vi "AMC_select_IP_SubVI.vi"(10 "IPs":string[](array[string]), 11 "Found Devices":T1(array[cluster])) -> (0 "error out":errorcluster, 2 "Device Info":T2, 3 "IP":string)   [LabVIEW 2019]
panel:
  out "Found devices":i32
  in  "please select IP":u16(ring) items=["10.10.1.230", "192.168.1.1"]
  in  "Refresh Button":bool
  in  "Process Stop":bool
  in  "OK Button":bool
  out "Array":T1(array[cluster])
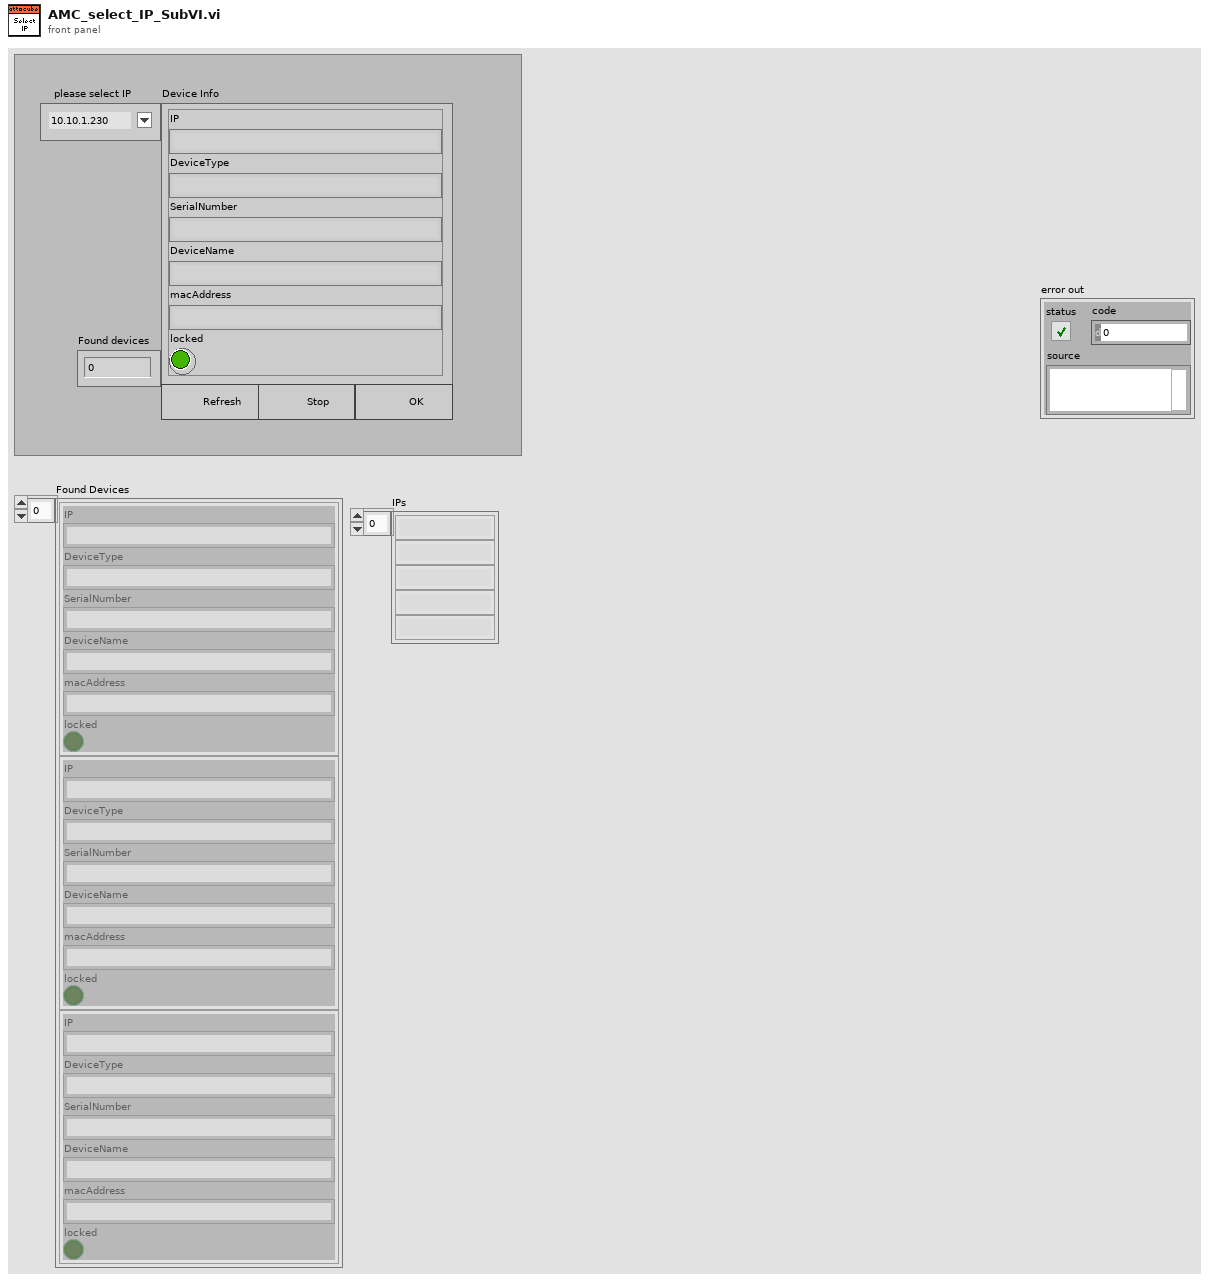
[diagram p1: front panel]
types:
  T1 = cluster{"IP":string, "DeviceType":string, "SerialNumber":string, "DeviceName":string, "macAddress":string, "locked":bool}[]
  T2 = cluster{"IP":string, "DeviceType":string, "SerialNumber":string, "DeviceName":string, "macAddress":string, "locked":bool}
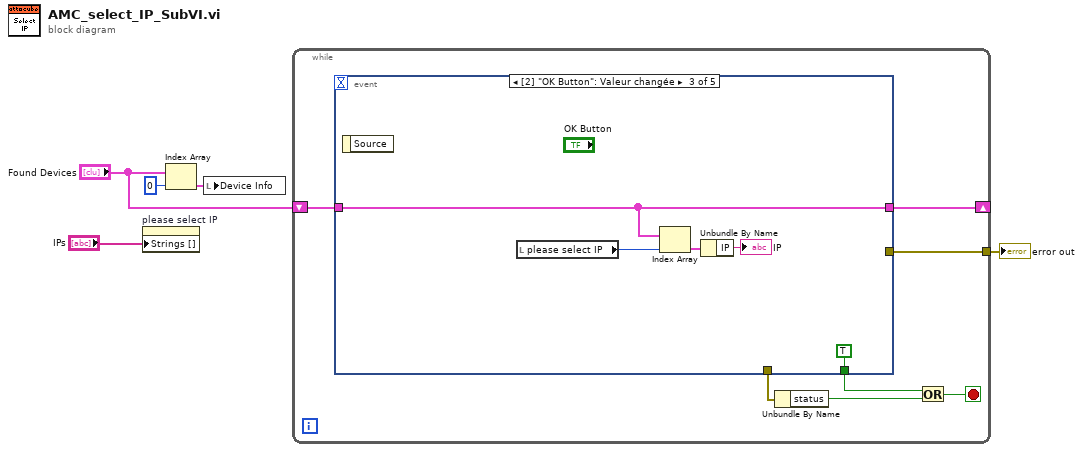
[diagram p0: block diagram]
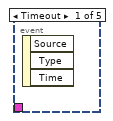
[diagram p2: hidden frame]
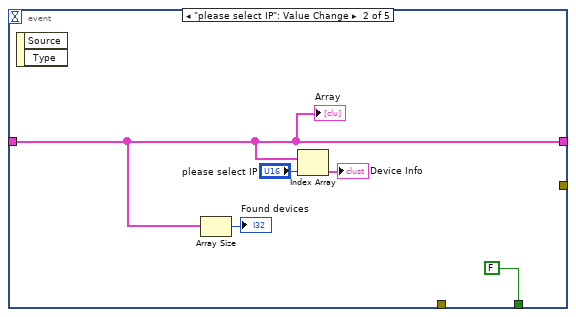
[diagram p3: hidden frame]
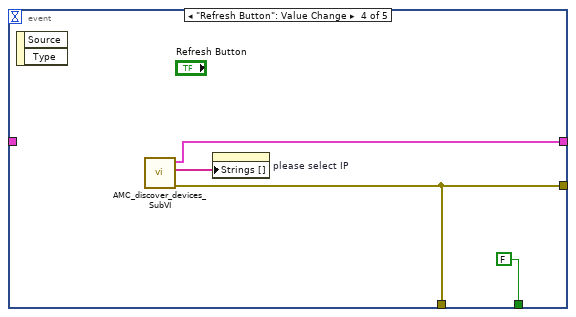
[diagram p4: hidden frame]
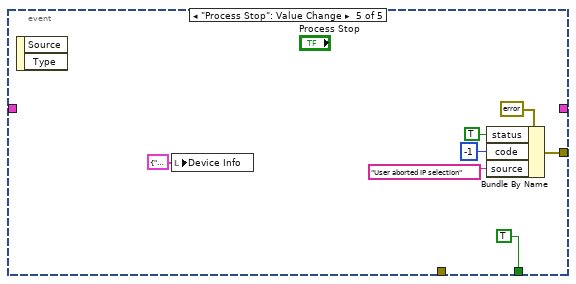
[diagram p5: hidden frame]
diagram:
  n1 = property on="please select IP" class="MDér (strict)"("Strings []"="IPs") -> ()  [unwired: 2 in, 2 out]
  n2 = Index Array(array="Found Devices", index=0) -> (element=w3:T2)
  n3 = local write "Device Info"(w3) -> ()
  n4 = while {
    shift-right: [w12] -> _
    shift-left: "Found Devices" -> [w11]
    tunnel: [w6] -> w5
    stop <- w7 stop-if-true
    n5 = event shown="[2] \"OK Button\": Valeur changée" {
      selector: _ -> [_ _ _ _ _]
      dyn-events: _ -> [_ _ _ _ _]
      timeout: _ -> [_ _ _ _ _]
      tunnel: [_ w14 w20 w25 _] -> w12
      tunnel: w11 -> [_ w14 w20 _ _]
      tunnel: [_ FALSE TRUE FALSE TRUE] -> w9
      tunnel: [_ _ _ w23 _] -> w10
      tunnel: [_ _ _ w23 w27] -> w6
      event Timeout {
        n6 = event-data() -> ()  [unwired: 1 in, 3 out]
      }
      event "please select IP": Value Change {
        n7 = event-data() -> ()  [unwired: 1 in, 2 out]
        n8 = Array Size(array=w14) -> (size(s)=→"Found devices":i32)
        n9 = Index Array(array=w14, index="please select IP") -> (element=→"Device Info":T2)
        "Array" <- w14
      }
      event "OK Button": Value Change {
        n10 = event-data() -> ()  [unwired: 1 in, 1 out]
        n11 = local read "please select IP"() -> (w18:u16)
        n12 = Index Array(array=w20, index=w18) -> (element=w21:T2)
        n13 = Unbundle By Name(w21) -> ("IP"=→"IP":string)
      }
      event "Refresh Button": Value Change {
        n14 = event-data() -> ()  [unwired: 1 in, 2 out]
        n15 = call <userlib>:"AMC_discover_devices_SubVI.vi"() -> ("error out"=w23:errorcluster, "IPs"=w26:string[], "Found Devices"=w25:T1)  [unwired: 8 in, 1 out]
        n16 = property on="please select IP" class="MDér (strict)"("Strings []"=w26) -> ()  [unwired: 2 in, 2 out]
      }
      event "Process Stop": Value Change {
        n17 = event-data() -> ()  [unwired: 1 in, 2 out]
        n18 = local write "Device Info"(T2 {"IP"="", "DeviceType"="", "SerialNumber"="", "DeviceName"="", "macAddress"="", "locked"=FALSE} ("Cluster")) -> ()
        n19 = Bundle By Name(cluster=errorcluster {"status"=FALSE, "code"=0, "source"=""} ("error out"), "status"=TRUE, "code"=-1, "source"="User aborted IP selection") -> (w27:errorcluster)
      }
    }
    n20 = Unbundle By Name(w10) -> ("status"=w8:bool)
    n21 = Or(x=w9, y=w8) -> (x .or. y?=w7:bool)
  }
  "error out" <- w5
